vi "GEA2 Script_Log Report.vi"(0 "Test failures":string, 5 "Log File Path":path, 7 "Header":string, 11 "Error In":errorcluster, 13 "Script":string) -> (15 "Error Out":errorcluster)   [LabVIEW 2016]
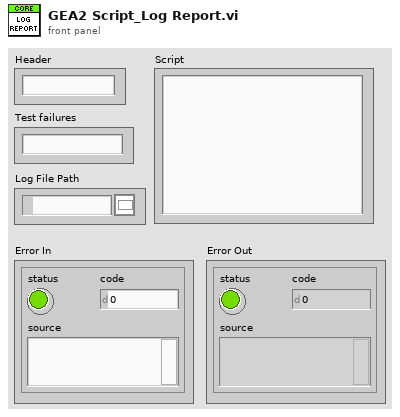
[diagram p1: front panel]
types:
  T1 = enum16{"open", "replace", "create", "open or create", "replace or create", "replace or create with confirmation"}
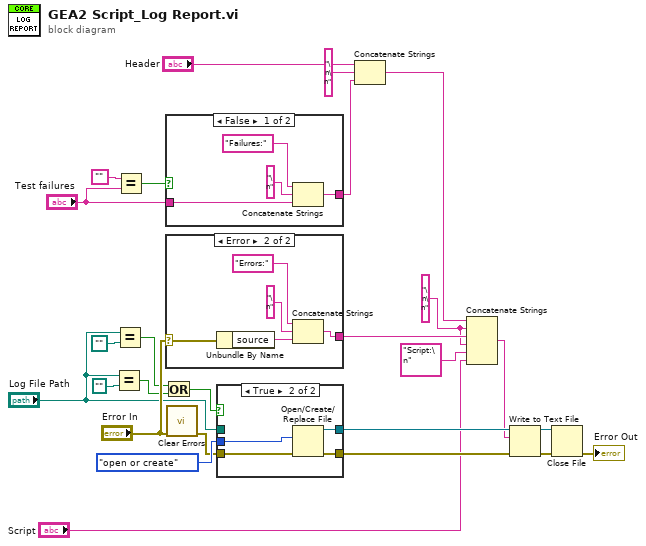
[diagram p0: block diagram]
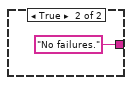
[diagram p2: hidden frame]
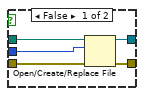
[diagram p3: hidden frame]
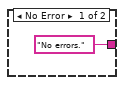
[diagram p4: hidden frame]
diagram:
  w3 = "\n\n" ("string")
  n1 = Equal?(x="Log File Path", y=path "") -> (x = y?=w13:bool)
  n2 = Equal?(x="Log File Path", y=path "") -> (x = y?=w12:bool)
  n3 = Equal?(x="", y="Test failures") -> (x = y?=w9:bool)
  n4 = Or(x=w12, y=w13) -> (x .or. y?=w11:bool)
  n5 = case shown="False" w9 {
    tunnel: [w27 "No failures." ("String")] -> w7
    tunnel: "Test failures" -> [w28 _]
    frame False {
      n6 = Concatenate Strings("Failures:" ("string"), "\n" ("string"), w28) -> (w27:string)
    }
    frame True {
    }
  }
  n7 = case shown="Error" "Error In" {
    selector: "Error In" -> [_ w37]
    tunnel: ["No errors." w35] -> w17
    frame No Error {
    }
    frame Error {
      n8 = Unbundle By Name(w37) -> ("source"=w36:string)
      n9 = Concatenate Strings("Errors:" ("string"), "\n" ("string"), w36) -> (w35:string)
    }
  }
  n10 = call <vilib>:"Clear Errors.vi"("error in (no error)"="Error In") -> ("error out"=w18:errorcluster)  [unwired: 5 in, 1 out]
  n11 = case shown="True" w11 {
    tunnel: [w41 w46] -> w25
    tunnel: [w40 w45] -> w24
    tunnel: T1."open or create" ("operation (0:open)") -> [w38 w44]
    tunnel: w18 -> [w42 w43]
    tunnel: "Log File Path" -> [w39 _]
    frame False {
      n12 = Open/Create/Replace File(file path (use dialog)=w39, error in=w42, operation (0:open)=w38) -> (refnum out=w40:refnum<file>, error out=w41:errorcluster)  [unwired: 3 in, 1 out]
    }
    frame True {
      n13 = Open/Create/Replace File(error in=w43, operation (0:open)=w44) -> (refnum out=w45:refnum<file>, error out=w46:errorcluster)  [unwired: 4 in, 1 out]
    }
  }
  n14 = Concatenate Strings("Header", "\n\n" ("string"), w7) -> (w6:string)
  n15 = Concatenate Strings(w6, w3, w17, w3, "Script:\n" ("string"), "Script") -> (w20:string)
  n16 = Write to Text File(file (use dialog)=w24, text=w20, error in=w25) -> (refnum out=w23:refnum<file>, error out=w26:errorcluster)  [unwired: 1 in, 1 out]
  n17 = Close File(refnum=w23, error in=w26) -> (error out=→"Error Out":errorcluster)  [unwired: 1 out]
